vi "Drive_Set.vi"   [LabVIEW 2019]
uses:
  DriveExecuteCluster.ctl
  Drive_Globals.vi
types:
  T1 = typedef "DriveExecuteCluster.ctl" = cluster{"Front/Back":dbl, "Turn":dbl, "Drive Control Type":enum16{"PercentVoltage", "SpeedControl"}}
  T2 = typedef "DriveSetCluster.ctl" = cluster{"Front/Back":dbl, "Turn":dbl, "Speed_Control?":bool}
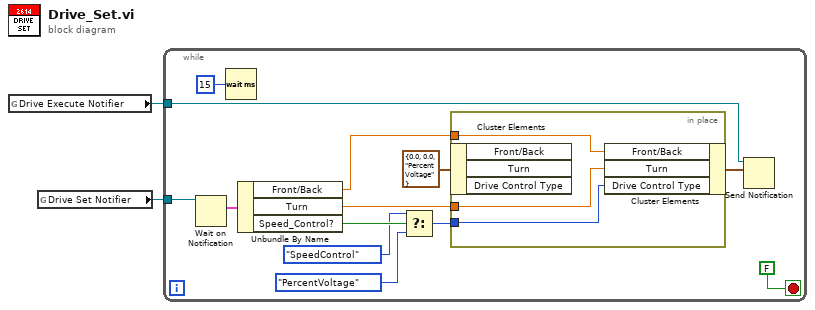
[diagram p0: block diagram]
diagram:
  n1 = global read "Drive_Globals.vi" "Drive Execute Notifier"() -> (w1:refnum<notifier>)
  n2 = global read "Drive_Globals.vi" "Drive Set Notifier"() -> (w2:refnum<notifier>)
  n3 = while {
    tunnel: w2 -> [w14]
    tunnel: w1 -> [w12]
    stop <- FALSE stop-if-true
    n4 = Wait on Notification(notifier=w14) -> (notification=w13:T2)  [unwired: 3 in, 3 out]
    n5 = Wait (ms)(milliseconds to wait=u32 15) -> ()  [unwired: 1 out]
    n6 = Unbundle By Name(w13) -> ("Front/Back"=w5:dbl, "Turn"=w4:dbl, "Speed_Control?"=w11:bool)
    n7 = Select(t=enum16{"PercentVoltage", "SpeedControl"}."SpeedControl" ("Drive Control Type"), s=w11, f=enum16{"PercentVoltage", "SpeedControl"}."PercentVoltage" ("Drive Control Type")) -> (s? t:f=w3:enum16{"PercentVoltage", "SpeedControl"})
    n8 = in-place {
      in-place-border: w5 -> [w18]
      in-place-border: w4 -> [w17]
      in-place-border: w3 -> [w16]
      n9 = in-place-cluster #1(T1 {"Front/Back"=0.0, "Turn"=0.0, "Drive Control Type"=enum."PercentVoltage"} ("notification")) -> ()  [unwired: 3 out]
      n10 = in-place-cluster #1("Front/Back"=w18, "Turn"=w17, "Drive Control Type"=w16) -> (w6:T1)
    }
    n11 = Send Notification(notification=w6, notifier=w12) -> ()  [unwired: 1 in, 2 out]
  }
